vi "Test Handle Results is Called.vi"(8 "error in (no error)":errorcluster, 11 "XML Report Test in":refnum<class "Report Generator Test.lvclass">) -> (0 "error out":errorcluster, 3 "XML Report Test out":refnum<class "Report Generator Test.lvclass">)   [LabVIEW 2020, in "Report Generator Test.lvclass"]
uses:
  Report Generator Test.lvclass
  Report Generator Test.lvclass/Report Generator Test.ctl
  Test Doubles/Mock Report/Mock Report.lvclass
  7fd9b121-f230-4a1e-b835-77146010e6b9.vi
  source/Core/Result/Status.ctl
  source/Core/Result/Result.lvlib
  source/Core/Result/Type.ctl
  source/Core/Result/Result.ctl
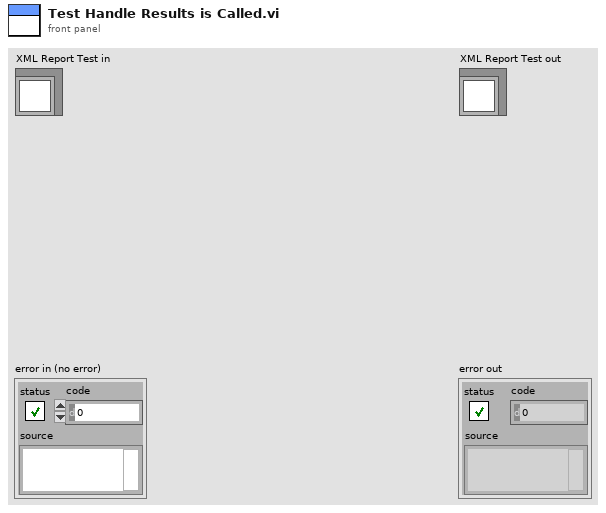
[diagram p1: front panel]
types:
  T1 = typedef "Result.lvlib/Result.ctl" = cluster{"Name":string, "Description":string, "Status":T2, "Result Type":T3, "Execution Time":dbl, "Data":cluster{"Expected":variant, "Actual":variant, "Delta":variant}}
  T2 = typedef "Result.lvlib/Status.ctl" = enum16{"", "Passed", "Failed", "Error", "Skipped", "Setup Error", "Broken", "Teardown Error"}
  T3 = typedef "Result.lvlib/Type.ctl" = enum16{"Test Case", "Test Suite", "Test Run", "Pass", "Fail", "Skip", "Pass if", "Fail if", "Pass if Error", "Fail if Error", "Pass if Equal", "Fail if Equal"}
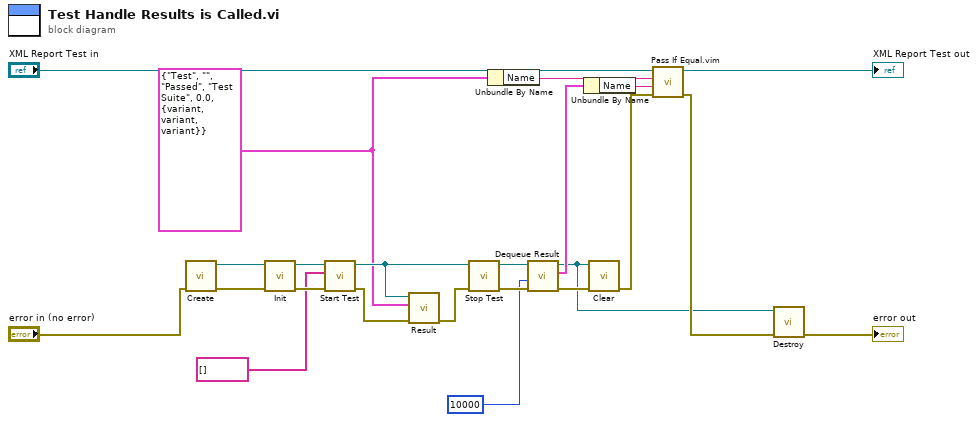
[diagram p0: block diagram]
diagram:
  w10 = T1 {"Name"="Test", "Description"="", "Status"=enum."Passed", "Result Type"=enum."Test Suite", "Execution Time"=0.0, "Data"={"Expected"=variant, "Actual"=variant, "Delta"=variant}} ("Result")
  n1 = call "Create.vi"("error in (no error)"="error in (no error)") -> ("error out"=w7:errorcluster, "Mock Report Out"=w9:refnum<class "Mock Report.lvclass">)  [unwired: 9 in]
  n2 = call-dynamic "Init.vi"("error in (no error)"=w7, "Mock Report In"=w9) -> ("error out"=w19:errorcluster, "Mock Report Out"=w20:refnum<class "Mock Report.lvclass">)  [unwired: 8 in]
  n3 = call-dynamic "Start Test.vi"("error in (no error)"=w19, "Tests"=string[] [], "XML Report in"=w20) -> ("error out"=w18:errorcluster, "XML Report out"=w16:refnum<class "Mock Report.lvclass">)  [unwired: 7 in]
  n4 = call-dynamic "Result.vi"("error in (no error)"=w18, "Result"=w10, "Report In"=w16) -> ("error out"=w17:errorcluster)  [unwired: 8 in]
  n5 = call-dynamic "Stop Test.vi"("error in (no error)"=w17, "XML Report in"=w16) -> ("error out"=w14:errorcluster, "XML Report out"=w15:refnum<class "Mock Report.lvclass">)  [unwired: 8 in]
  n6 = Unbundle By Name(w10) -> ("Name"=w2:string)
  n7 = call "Dequeue Result.vi"("error in (no error)"=w14, "timeout in ms (0)"=10000, "Mock Report In"=w15) -> ("error out"=w13:errorcluster, "Result"=w11:T1, "Mock Report Out"=w5:refnum<class "Mock Report.lvclass">)  [unwired: 6 in]
  n8 = Unbundle By Name(w11) -> ("Name"=w3:string)
  n9 = call-dynamic "Clear.vi"("error in (no error)"=w13, "XML Report in"=w5) -> ("error out"=w12:errorcluster)  [unwired: 9 in]
  n10 = call "Pass If Equal.vim"("error in (no error)"=w12, "Actual"=w3, "Expected"=w2, "LUnit Test Case In"="XML Report Test in") -> ("error out"=w21:errorcluster, "LUnit Test Case Out"=→"XML Report Test out":refnum<class "Report Generator Test.lvclass">)  [unwired: 6 in]
  n11 = call "Destroy.vi"("error in (no error)"=w21, "Mock Report In"=w5) -> ("error out"=→"error out":errorcluster)  [unwired: 9 in]
